vi "DSF.Shared.Configuration.Transfer.Initialize.vi"(7 "Custom Parameters":variant, 8 "error in (no error)":errorcluster, 9 "Channel Descriptors":T1[](array[typedef]) {"VS Channel Ref" format="%016x"; "Channel Parameters"."offset" format="%d bytes"}, 10 "Name":string, 11 "Transfer Configuration in":refnum<class "DSF.Shared.Configuration.Transfer.lvclass">) -> (0 "error out":errorcluster, 3 "Transfer Configuration out":refnum<class "DSF.Shared.Configuration.Transfer.lvclass">)   [LabVIEW 2017, in "DSF.Shared.lvlib" / "DSF.Shared.Configuration.Transfer.lvclass"]
uses:
  DSF.Shared.Configuration.Transfer.lvclass
  Configuration/DSF.Shared.Configuration.lvclass
  C:/Git/Sourcetree/DSF/Source/Shared/Classes/Configuration/DSF.Shared.Configuration.lvclass
  Typedefs/DSF.Shared.Typedefs.Data Type.ctl
  DSF.Shared.lvlib
  Typedefs/DSF.Shared.Typedefs.Configuration.Transfer.Channel Descriptor.ctl
  <vilib>/NI Veristand/Custom Device API/Custom Device Item Ref.ctl
  <vilib>/NI Veristand/Custom Device API/Custom Device API.lvlib
  Typedefs/DSF.Shared.Typedefs.Configuration.Transfer.Channel Parameters.ctl
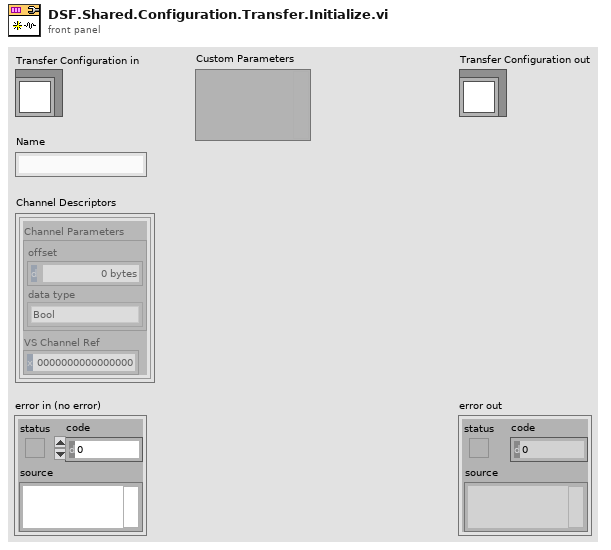
[diagram p1: front panel]
types:
  T1 = typedef "DSF.Shared.lvlib/DSF.Shared.Typedefs.Configuration.Transfer.Channel Descriptor.ctl" = cluster{"Channel Parameters":T2, "VS Channel Ref":T4}
  T2 = typedef "DSF.Shared.lvlib/DSF.Shared.Typedefs.Configuration.Transfer.Channel Parameters.ctl" = cluster{"offset":u64, "data type":T3}
  T3 = typedef "DSF.Shared.lvlib/DSF.Shared.Typedefs.Data Type.ctl" = enum8{"Bool", "SGL", "DBL", "I8", "I16", "I32", "I64", "U8", "U16", "U32", "U64"}
  T4 = typedef "Custom Device API.lvlib/Custom Device Item Ref.ctl" = u64
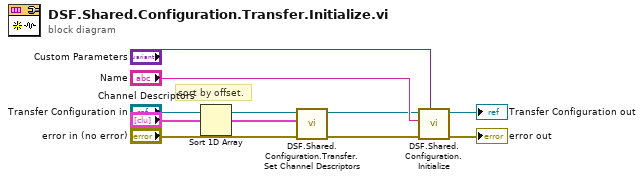
[diagram p0: block diagram]
diagram:
  # "sort by offset."
  n1 = Sort 1D Array(array="Channel Descriptors") -> (sorted array=w7:T1[])
  n2 = call "DSF.Shared.Configuration.Transfer.Set Channel Descriptors.vi"("Channel Descriptors"=w7, "Transfer Configuration in"="Transfer Configuration in") -> ("Transfer Configuration out"=w1:refnum<class "DSF.Shared.Configuration.Transfer.lvclass">)  [unwired: 9 in]
  n3 = call "DSF.Shared.Configuration.Initialize.vi"(7:"Custom Parameters", "error in (no error)"="error in (no error)", "name"="Name", "Configuration in"=w1) -> ("error out"=→"error out":errorcluster, "Configuration out"=→"Transfer Configuration out":refnum<class "DSF.Shared.Configuration.Transfer.lvclass">)  [unwired: 6 in]
